vi "Binary Serialise Complex DBL Vector.vi"(7 "Expected Class":refnum<class "Var_CPLX_DBL.lvclass">, 8 "error in (no error)":errorcluster, 11 "Test Value":cdb) -> (0 "error out":errorcluster)   [LabVIEW 2021]
uses:
  Source/Variables/Support/CPLX_DBL/Var_CPLX_DBL.lvclass
  C:/TSA/LV_Abstract/Source/Abs_Types/Complex Double Float/Abs_Complex Double Float.lvclass
  Source/Variables/Support/CPLX_DBL/Support/Init_Simple_Var.vi
  Source/Abs_Types/Complex Double Float/Simple Read.vi
  <vilib>/addons/_JKI Toolkits/Caraya/classes/Assert/Assert Equal Value_Variant.vi
  <vilib>/addons/_JKI Toolkits/Caraya/classes/Assert/Assert Equal Type_Variant.vi
  <vilib>/addons/_JKI Toolkits/Caraya/classes/Assert/Assert.lvclass
  <vilib>/addons/_JKI Toolkits/Caraya/classes/Test/Test.lvclass
  <vilib>/Utility/Data Type/NI_Data Type.lvlib
  Source/Abs_Types/Complex Double Float/Abs_Complex Double Float.lvclass
  C:/TSA/LV_Abstract/Source/Abs_Types/Floating Point/Abs_Floating Point.lvclass
  C:/Program Files (x86)/National Instruments/LabVIEW 2021/vi.lib/TSA/Abstract Data Classes/Abs_Types/Numeric/Abs_Numeric.lvclass
  C:/Program Files (x86)/National Instruments/LabVIEW 2021/vi.lib/TSA/Abstract Data Classes/Abs_Types/Value/Abs_Value.lvclass
  C:/Program Files (x86)/National Instruments/LabVIEW 2021/vi.lib/TSA/Abstract Data Classes/Abs_Types/Type/Abs_Type.lvclass
  C:/TSA/LV_Abstract/Source/Variables/Support/CPLX_DBL/Var_CPLX_DBL.lvclass
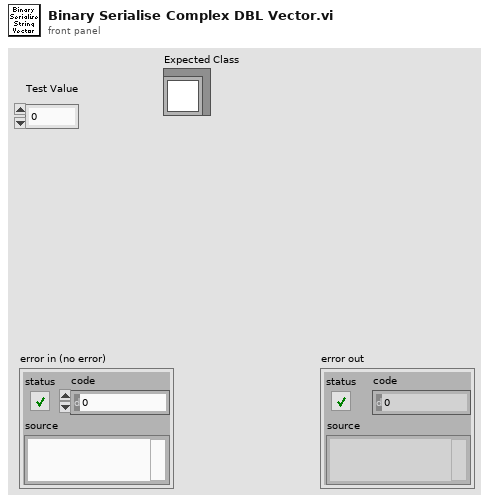
[diagram p1: front panel]
types:
  T1 = typedef "NI_Data Type.lvlib/Data Type.ctl" = enum8{"Invalid Type", "Void", "I8", "I16", "I32", "I64", "U8", "U16", "U32", "U64", "Single Float", "Double Float", "Extended Float", "Single Complex", "Double Complex", "Extended Complex", "Enum U8", "Enum U16", "Enum U32", "Enum U64", "Single Float With Unit", "Double Float With Unit", "Extended Float With Unit", "Single Complex with Unit", "Double Complex with Unit", "Extended Complex with Unit", "Boolean", "String", "Path", "Picture", "Tag", "Array", "Cluster", "Variant", "LV Variant", "Waveform", "Timestamp", "Digital Waveform", "Digital Data", "ExpressData", "Refnum", "External Data", "VI", "Poly VI", "LabVIEW Class Instance", "Fixed Point", "Set Collection", "Map Collection"}
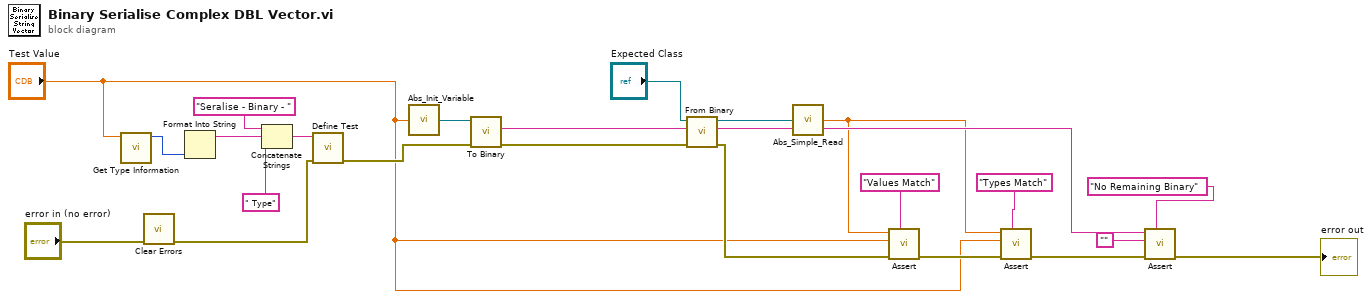
[diagram p0: block diagram]
diagram:
  n1 = call <vilib>:"Get Type Information.vi"("variant"="Test Value") -> ("type"=w15:T1)  [unwired: 6 in, 4 out]
  n2 = call <vilib>:"Clear Errors.vi"("error in (no error)"="error in (no error)") -> ("error out"=w10:errorcluster)  [unwired: 5 in, 1 out]
  n3 = Format Into String(w15) -> (resulting string=w14:string)  [unwired: 3 in, 1 out]
  n4 = Concatenate Strings("Seralise - Binary - " ("string"), w14, " Type" ("string")) -> (w13:string)
  n5 = call <vilib>:"Define Test.vi"("error in (no error)"=w10, "Label (VI Title)"=w13) -> ("error out"=w4:errorcluster)  [unwired: 8 in, 1 out]
  n6 = call-poly "Abs_Init_Variable.vi"("Value"="Test Value") -> ("Var"=w3:refnum<class "Var_CPLX_DBL.lvclass">)  [unwired: 4 in]
  n7 = call-dynamic "To Binary.vi"("error in (no error)"=w4, "Double Float in"=w3) -> ("error out"=w23:errorcluster, "Binary"=w24:string)  [unwired: 7 in, 1 out]
  n8 = call-dynamic "From Binary.vi"("error in (no error)"=w23, "Binary"=w24, "Double Float in"="Expected Class") -> ("error out"=w21:errorcluster, "Remaining"=w19:string, "Double Float out"=w22:refnum<class "Var_CPLX_DBL.lvclass">)  [unwired: 6 in]
  n9 = call-poly "Abs_Simple_Read.vi"("Class"=w22) -> ("Value"=w7:cdb)  [unwired: 4 in]
  n10 = call-poly <vilib>:"Assert.vi"("Label"="Values Match", "error in (no error)"=w21, "Actual"="Test Value", "Expected"=w7) -> ("error out"=w8:errorcluster)  [unwired: 6 in, 1 out]
  n11 = call-poly <vilib>:"Assert.vi"("Label"="Types Match", "error in (no error)"=w8, "Actual"="Test Value", "Expected"=w7) -> ("error out"=w6:errorcluster)  [unwired: 6 in, 1 out]
  n12 = call-poly <vilib>:"Assert.vi"("Label"="No Remaining Binary", "error in (no error)"=w6, "Actual"="", "Expected"=w19) -> ("error out"=→"error out":errorcluster)  [unwired: 6 in, 1 out]
